vi "Demo_AddSoundToMovie.vi"(9 "Insert where [in movie timescale]":i32=1000, 10 "Movie file path":path=path "/BootX/Users/chris/Desktop/AddSoundToMovie/GdPapa.mov", 11 "Sound file path":path=path "/BootX/Users/chris/Desktop/AddSoundToMovie/10SecWavSound.wav") -> ()   [LabVIEW 2024]
doc: "Add the sound tracks of the sound file to the movie file.\nThe movie file is overwritten (make a copy if you want to keep the original)\nThe movie file is flattened to improve playback performances.\nA temporary file is created since it is not always possible to do these opereations in place.\n\nIT MAY TAKES TIME, be patient!\n\n © Chris Salzmann 1994 - 2003"
uses:
  <userlib>/ImageProcessing/QTLIB_2595_LV86/QT_File.ctl
  <userlib>/ImageProcessing/QTLIB_2595_LV86/QT_Sound.ctl
  <userlib>/ImageProcessing/QTLIB_2595_LV86/QT_Private.ctl
panel:
  out "error out":errorcluster={"status"=TRUE, "code"=-47, "source"="kAddSoundToMovie"}
  # "Add the sound tracks of the sound file to the movie file.\nThe movie file is overwritten (make a copy if you want to keep the original)\nThe movie file is flattened to improve playback performances.\nA temporary file is created since it is not always possible to do these opereations in place.\n\nIT MAY TAKES TIME, be patient!\n\n © Chris Salzmann 1994 - 2005"
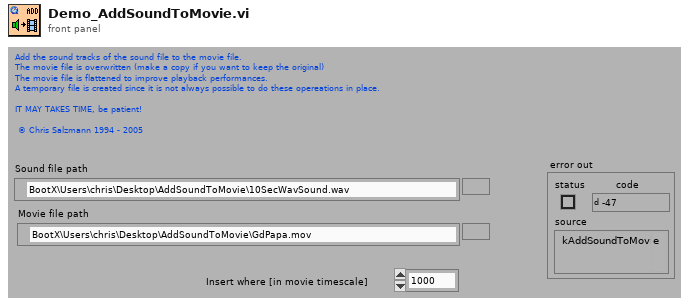
[diagram p1: front panel]
types:
  T1 = typedef "QT_Private.ctl" = cluster{"reserved 1":i32, "reserved 2":i32, "reserved 3":i32, "reserved 4":i32}
  T2 = typedef "QT_Sound.ctl" = cluster{"Nbr samples":i32, "Samples size":i32, "Nbr channels":i32, "Rate ":i32, "Compression":i32, "Codec":string, "Vendor":string, "Quality":i32, "data":i16[], "Compressed data":u8[], "Duration":i32, "Position":i32, "Options":i32, "Reserved":i32}
  T3 = typedef "QT_File.ctl" = cluster{"Paths":string[], "Options":i32, "Dialogs":u32, "Reserved":i32}
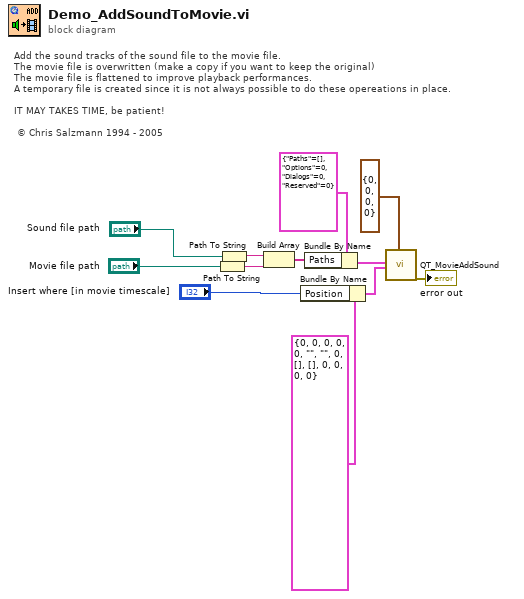
[diagram p0: block diagram]
diagram:
  # "Add the sound tracks of the sound file to the movie file.\nThe movie file is overwritten (make a copy if you want to keep the original)\nThe movie file is flattened to improve playback performances.\nA temporary file is created since it is not always possible to do these opereations in place.\n\nIT MAY TAKES TIME, be patient!\n\n © Chris Salzmann 1994 - 2005"
  n1 = Path To String(path="Movie file path") -> (string=w9:string)
  n2 = Path To String(path="Sound file path") -> (string=w10:string)
  n3 = Build Array(w10, w9) -> (w4:string[])
  n4 = Bundle By Name(cluster=T2 {"Nbr samples"=0, "Samples size"=0, "Nbr channels"=0, "Rate "=0, "Compression"=0, "Codec"="", "Vendor"="", "Quality"=0, "data"=[], "Compressed data"=[], "Duration"=0, "Position"=0, "Options"=0, "Reserved"=0} ("Sound in"), "Position"="Insert where [in movie timescale]") -> (w2:T2)
  n5 = Bundle By Name(cluster=T3 {"Paths"=[], "Options"=0, "Dialogs"=0, "Reserved"=0} ("File Settings"), "Paths"=w4) -> (w3:T3)
  n6 = call <userlib>:"QT_MovieAddSound.vi"("File Settings"=w3, "Sound in"=w2, "Private"=T1 {"reserved 1"=0, "reserved 2"=0, "reserved 3"=0, "reserved 4"=0}) -> ("error out"=→"error out":errorcluster)  [unwired: 2 in, 14 out]
